vi "量程判断-未完成.vi"   [LabVIEW 2019]
uses:
  lib/Stanford Research 830/Stanford Research 830.lvlib
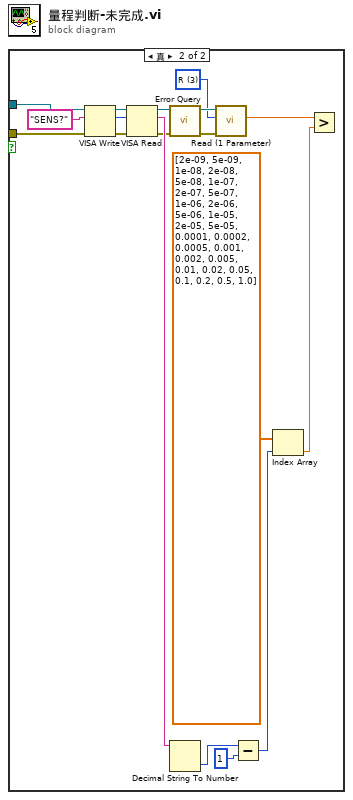
[diagram p0: block diagram]
diagram:
  n1 = case shown="真" {
    selector: _ -> [_ _]
    tunnel: _ -> [_ w15]
    tunnel: _ -> [_ w14]
    frame False {
    }
    frame True {
      w1 = u16 3 items=["X"=1, "Y"=2, "R"=3, "Theta"=4, "Channel 1"=5, "Channel 2"=6, "Aux In 1"=7, "Aux In 2"=8, "Aux In 3"=9, "Aux In 4"=10] ("Parameter (1: X)")
      n2 = VISA Write(VISA resource name=w15, write buffer="SENS?" ("写入缓冲区"), error in (no error)=w14) -> (VISA resource name out=w18:refnum<visa-resource-name>, return count=w16:u32, error out=w17:errorcluster)
      n3 = VISA Read(VISA resource name=w18, byte count=w16, error in (no error)=w17) -> (VISA resource name out=w5:refnum<visa-resource-name>, read buffer=w12:string, error out=w4:errorcluster)  [unwired: 1 out]
      n4 = call "Error Query.vi"("error in (no error)"=w4, "VISA resource name"=w5) -> ("error out"=w2:errorcluster, "VISA resource name out"=w3:refnum<visa-resource-name>)  [unwired: 7 in, 1 out]
      n5 = Decimal String To Number(string=w12) -> (number=w10:i32)  [unwired: 2 in, 1 out]
      n6 = call "Read (1 Parameter).vi"("error in (no error)"=w2, "Parameter (1: X)"=w1, "VISA resource name"=w3) -> ("Measurement"=w7:dbl)  [unwired: 6 in, 2 out]
      n7 = Subtract(x=w10, y=1) -> (x-y=w8:i32)
      n8 = Index Array(array=dbl[] [2e-09, 5e-09, 1e-08, 2e-08, 5e-08, 1e-07, 2e-07, 5e-07, 1e-06, 2e-06, 5e-06, 1e-05, 2e-05, 5e-05, 0.0001, 0.0002, 0.0005, 0.001, 0.002, 0.005, 0.01, 0.02, 0.05, 0.1, 0.2, 0.5, 1.0], index=w8) -> (element=w6:dbl)
      n9 = Greater?(x=w7, y=w6) -> ()  [unwired: 1 out]
    }
  }
